vi "Export_Spectra_To_Spreadsheet_File.vi"(4 "header? (write header:T)":bool=TRUE, 5 "delimiter (Tab)":string="\t", 6 "append to file? (new file:F)":bool, 7 "Array":cluster{"f0":dbl, "df":dbl, "magnitude":dbl[]}[](array[cluster]), 10 "file path (use dialog)":path) -> ()   [LabVIEW 2011]
doc: "Converts a waveform to a text string and writes the string to a new byte stream file or appends the string to an existing file. Wire data to the <B>Waveform</B> input to determine the polymorphic instance to use or manually select the instance."
uses:
  <vilib>/Waveform/WDTFileIO.llb/Export Waveforms To Spreadsheet File (1D).vi
panel:
  out "concatenated string":string
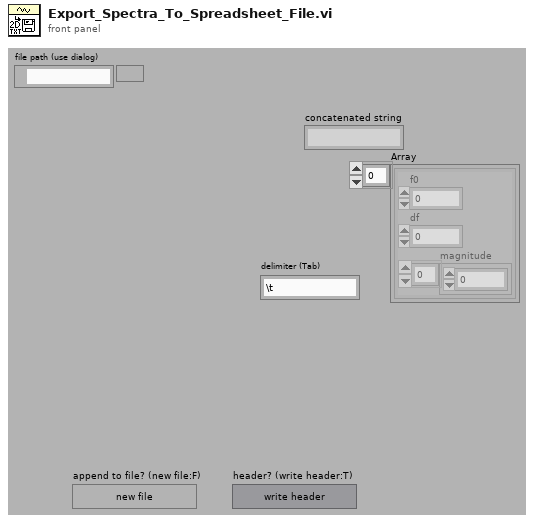
[diagram p1: front panel]
types:
  T1 = enum16{"open", "replace", "create", "open or create", "replace or create", "replace or create with confirmation"}
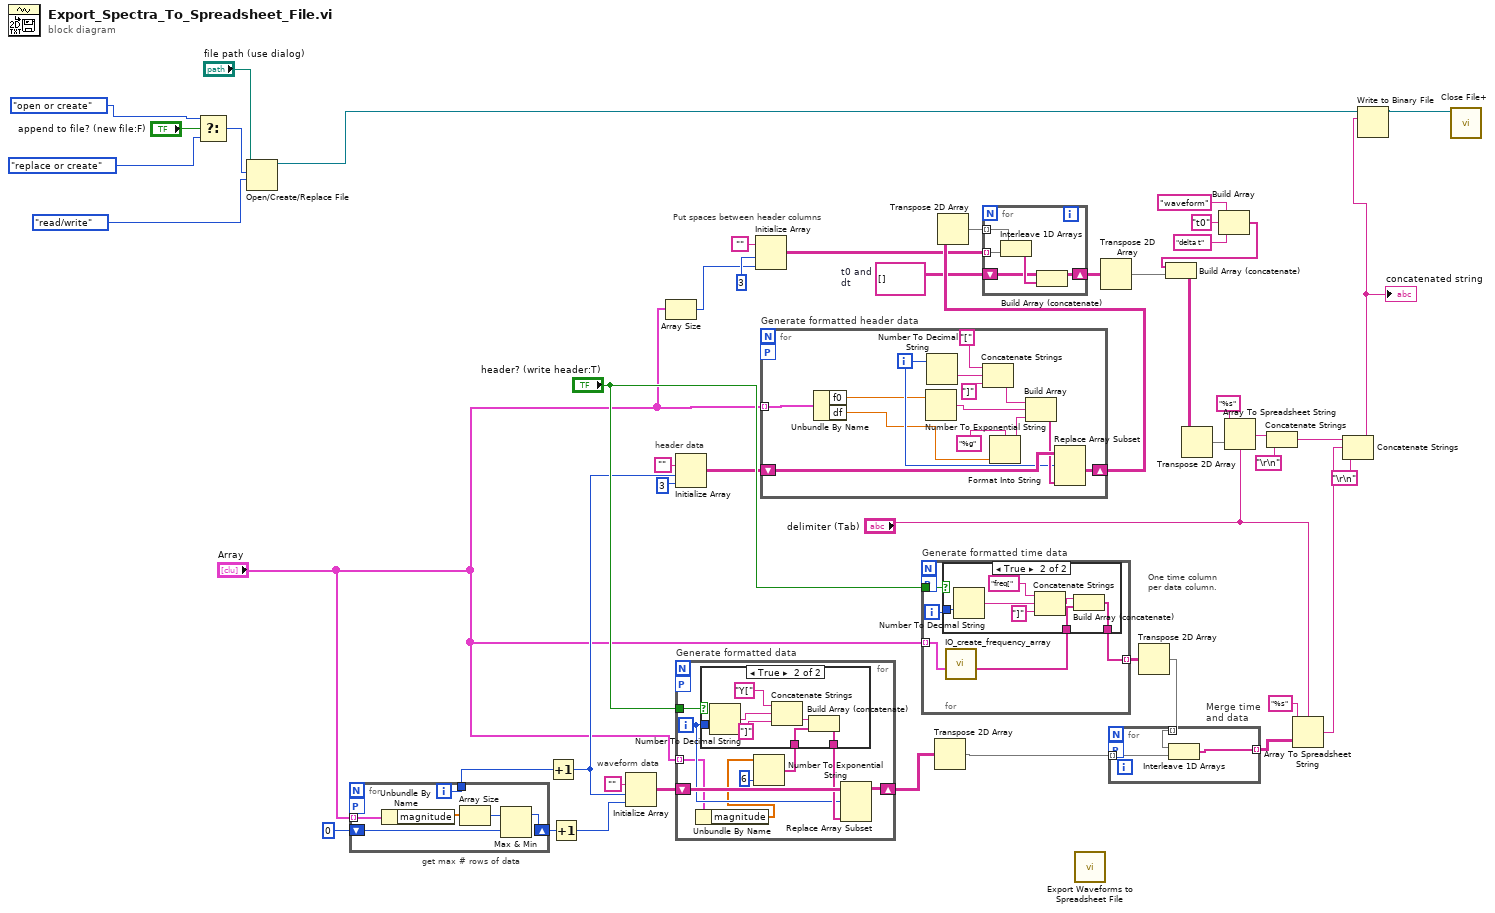
[diagram p0: block diagram]
diagram:
  w18 = string[][] []  # t0 and dt
  # "Put spaces between header columns"
  # "header data"
  # "One time column\nper data column."
  # "waveform data"
  # "get max # rows of data"
  n1 = Select ("function")(t=T1."open or create" ("operation (0:open)"), s="append to file? (new file:F)", f=T1."replace or create" ("operation (0:open)")) -> (s? t:f=w8:T1)
  n2 = Open/Create/Replace File(file path (use dialog)="file path (use dialog)", operation (0:open)=w8, access (0:read/write)=enum16{"read/write", "read-only", "write-only"}."read/write") -> (refnum out=w5:refnum<file>)  [unwired: 3 in, 2 out]
  n3 = for {
    tunnel: "Array" -> [w51] mode=indexing
    shift-right: [w53] -> w39
    shift-left: 0 -> [w54]
    tunnel: [w52] -> w40
    workers-P: _ -> [_]
    i -> [w52]
    n4 = Unbundle By Name(w51) -> ("magnitude"=w50:dbl[])
    n5 = Array Size(array=w50) -> (size(s)=w55:i32)
    n6 = Max & Min(x=w55, y=w54) -> (max(x,y)=w53:i32)  [unwired: 1 out]
  }
  n7 = Increment(x=w40) -> (x+1=w36:i32)
  n8 = Increment(x=w39) -> (x+1=w41:i32)
  n9 = Initialize Array("", w36, w41) -> (w35:string[][])
  n10 = Array Size(array="Array") -> (size(s)=w13:i32)
  n11 = Initialize Array("", w36, 3 ("dimension size")) -> (w21:string[][])
  n12 = for "Generate formatted data" {
    tunnel: "Array" -> [w57] mode=indexing
    shift-right: [w60] -> w45
    shift-left: w35 -> [w63]
    tunnel: "header? (write header:T)" -> [w62]
    workers-P: _ -> [_]
    i -> [w58]
    n13 = Unbundle By Name(w57) -> ("magnitude"=w56:dbl[])
    n14 = Number To Exponential String(number=w56, precision (6)=i16 6) -> (E-format string=w61:string[])  [unwired: 2 in]
    n15 = case shown="True" w62 {
      tunnel: w58 -> [_ w70]
      tunnel: w61 -> [w65 w68]
      tunnel: [w65 w67] -> w59
      frame False {
      }
      frame True {
        n16 = Number To Decimal String(number=w70) -> (decimal integer string=w72:string)  [unwired: 1 in]
        n17 = Concatenate Strings("Y[", w72, "]") -> (w69:string)
        n18 = Build Array (concatenate)(w69, w68) -> (w67:string[])
      }
    }
    n19 = Replace Array Subset(array=w63, new element=w59, index (row)=w58) -> (w60:string[][])  [unwired: 1 in]
  }
  n20 = Initialize Array("", 3 ("Dimension Size"), w13) -> (w17:string[][])
  n21 = for "Generate formatted header data" {
    shift-right: [w82] -> w20
    shift-left: w21 -> [w80]
    tunnel: "Array" -> [w77] mode=indexing
    workers-P: _ -> [_]
    i -> [w78]
    n22 = Unbundle By Name(w77) -> ("f0"=w75:dbl, "df"=w76:dbl)
    n23 = Number To Exponential String(number=w75) -> (E-format string=w74:string)  [unwired: 3 in]
    n24 = Number To Decimal String(number=w78) -> (decimal integer string=w84:string)  [unwired: 1 in]
    n25 = Concatenate Strings("[", w84, "]") -> (w85:string)
    n26 = Format Into String(format string="%g" ("Format String"), w76) -> (resulting string=w86:string)  [unwired: 2 in, 1 out]
    n27 = Build Array(w85, w74, w86) -> (w79:string[])
    n28 = Replace Array Subset(array=w80, new element=w79, index (row)=w78) -> (w82:string[][])  [unwired: 1 in]
  }
  n29 = for "Generate formatted time data" {
    tunnel: [w89] -> w34 mode=indexing
    tunnel: "Array" -> [w88] mode=indexing
    tunnel: "header? (write header:T)" -> [w90]
    workers-P: _ -> [_]
    i -> [w91]
    n30 = call "IO_create_frequency_array.vi"("cor"=w88) -> ("Array 2"=w87:string[])  [unwired: 10 in]
    n31 = case shown="True" w90 {
      tunnel: w91 -> [_ w97]
      tunnel: [w92 w94] -> w89
      tunnel: w87 -> [w92 w95]
      frame False {
      }
      frame True {
        n32 = Number To Decimal String(number=w97) -> (decimal integer string=w99:string)  [unwired: 1 in]
        n33 = Concatenate Strings("freq[", w99, "]") -> (w96:string)
        n34 = Build Array (concatenate)(w96, w95) -> (w94:string[])
      }
    }
  }
  n35 = Transpose 2D Array(2D array=w45) -> (transposed array=w12:string[][])
  n36 = Transpose 2D Array(2D array=w20) -> (transposed array=w15:string[][])
  n37 = for {
    shift-right: [w101] -> w16
    shift-left: w18 -> [w102]
    tunnel: w17 -> [w104] mode=indexing
    tunnel: w15 -> [w100] mode=indexing
    n38 = Interleave 1D Arrays(w100, w104) -> (w103:string[])
    n39 = Build Array (concatenate)(w102, w103) -> (w101:string[][])
  }
  n40 = call-poly <vilib>:"Export Waveforms to Spreadsheet File.vi"() -> ()  [unwired: 10 in, 2 out]
  n41 = Transpose 2D Array(2D array=w16) -> (transposed array=w26:string[][])
  n42 = Transpose 2D Array(2D array=w34) -> (transposed array=w11:string[][])
  n43 = for "Merge time\nand data" {
    tunnel: w12 -> [w107] mode=indexing
    tunnel: w11 -> [w106] mode=indexing
    tunnel: [w105] -> w10 mode=indexing
    workers-P: _ -> [_]
    n44 = Interleave 1D Arrays(w106, w107) -> (w105:string[])
  }
  n45 = Build Array("waveform", "t0", "delta t") -> (w27:string[])
  n46 = Build Array (concatenate)(w27, w26) -> (w24:string[][])
  n47 = Transpose 2D Array(2D array=w24) -> (transposed array=w25:string[][])
  n48 = Array To Spreadsheet String(delimiter (Tab)="delimiter (Tab)", array=w25, 3:"%s" ("format string")) -> (spreadsheet string=w29:string)
  n49 = Concatenate Strings(w29, "\r\n") -> (w46:string)
  n50 = Array To Spreadsheet String(delimiter (Tab)="delimiter (Tab)", array=w10, 3:"%s" ("format (%.3f)")) -> (spreadsheet string=w47:string)
  n51 = Concatenate Strings(w46, w47, "\r\n") -> (w3:string)
  "concatenated string" <- w3
  n52 = Write to Binary File(file (use dialog)=w5, data=w3) -> (refnum out=w4:refnum<file>)  [unwired: 4 in, 2 out]
  n53 = call <vilib>:"Close File+.vi"("refnum"=w4) -> ()  [unwired: 4 in, 3 out]
